vi "kalman measure step not single cycle.vi"(7 "vmax":fxp<+/-,32,0> format="%.32g", 10 "state in":T1={"pos estimate"=-30.139999389648438, "v estimate"=5.7999975979328156e-05, "weighted position error sum"=438.0, "photon count"=64, "transmit tick count"=0, "axis number"=0, "px (levels^2)"=298.0, "pxv (levels^2/ticks)"=0.003100000321865082, "pv (levels^2/ticks^2)"=6.199999802447564e-08, "vel diff (levels^2/ticks^3)"=0.0, "gx"=1.5546875, "rtwiddle"=66560.0}) -> (2 "state out":T1)   [LabVIEW 2010]
uses:
  integrating single axis kalman state.ctl
  <vilib>/rvi/FXPMathLib/FxpMul/XNode/nifxpmath_Multiplier.xnode
  <vilib>/rvi/FXPMathLib/FxpMul/subVIs/nifxpmath_Mul_SimConfig.ctl
  <vilib>/fxp/LVFixedPointQuantizationPolicyTypeDef.ctl
  <vilib>/fxp/LVFixedPointOverflowPolicyTypeDef.ctl
  <vilib>/rvi/FXPMathLib/FxpAdd/XNode/nifxpmath_Add.xnode
  <vilib>/rvi/FXPMathLib/FxpAdd/subVIs/nifxpmath_Add_SimConfig.ctl
  <vilib>/rvi/FXPMathLib/FxpReciprocal/XNode/nifxpmath_Reciprocal.xnode
  <vilib>/rvi/FXPMathLib/FxpDiv/XNode/nifxpmath_Div.xnode
  <vilib>/rvi/FXPMathLib/FxpDiv/subVIs/nifxpmath_Div_SimConfig.ctl
  <vilib>/rvi/FXPMathLib/FxpSub/XNode/nifxpmath_Sub.xnode
  <vilib>/rvi/FXPMathLib/FxpSub/subVIs/nifxpmath_Sub_SimConfig.ctl
  <vilib>/rvi/FXPMathLib/FxpMul/simVIs/DllFxpMulTemp_sub.vi
  <vilib>/rvi/FXPMathLib/FxpAdd/simVIs/DllFxpAddTemp_sub.vi
  <vilib>/rvi/FXPMathLib/FxpDiv/simVIs/DllFxpDivTemp_sub.vi
  <vilib>/rvi/FXPMathLib/FxpSub/simVIs/DllFxpSubTemp_sub.vi
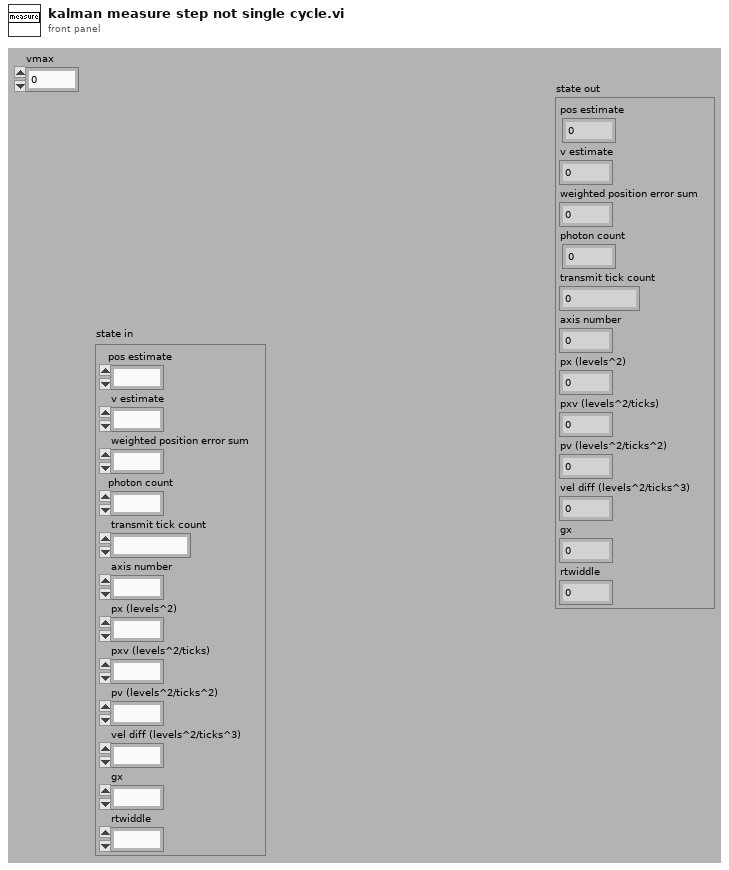
[diagram p1: front panel]
types:
  T1 = typedef "integrating single axis kalman state.ctl" = cluster{"pos estimate":fxp<+/-,32,16>, "v estimate":fxp<+/-,32,0>, "weighted position error sum":fxp<+/-,32,32>, "photon count":u32, "transmit tick count":u32, "axis number":u8, "px (levels^2)":fxp<+,32,19>, "pxv (levels^2/ticks)":fxp<+,32,2>, "pv (levels^2/ticks^2)":fxp<+,32,-14>, "vel diff (levels^2/ticks^3)":fxp<+,24,-22>, "gx":fxp<+,16,8>, "rtwiddle":fxp<+,16,26>}
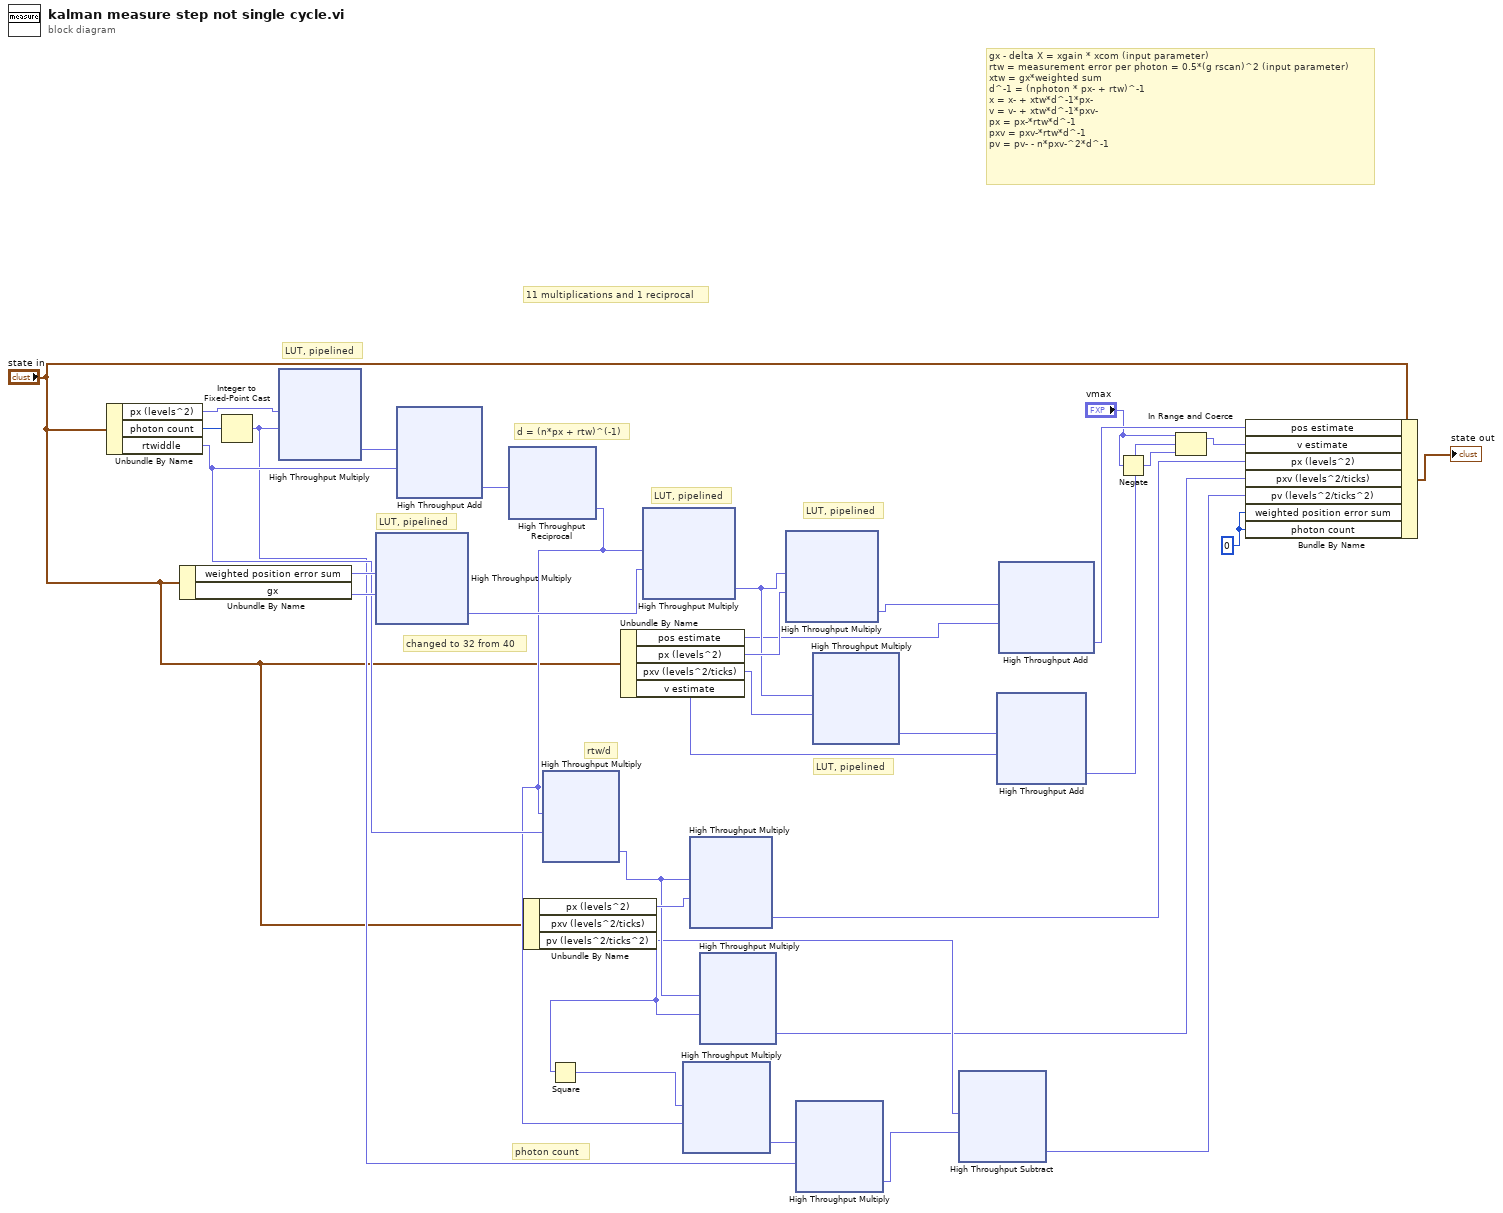
[diagram p0: block diagram]
diagram:
  w4 = i16 0
  # "LUT, pipelined"
  # "LUT, pipelined"
  # "changed to 32 from 40"
  # "LUT, pipelined"
  # "LUT, pipelined"
  # "LUT, pipelined"
  # "gx - delta X = xgain * xcom (input parameter)\nrtw = measurement error per photon = 0.5*(g rscan)^2 (input parameter)\nxtw = gx*weighted sum\nd^-1 = (nphoton * px- + rtw)^-1\nx = x- + xtw*d^-1*px-\nv = v- + xtw*d^-1*pxv-\npx = px-*rtw*d^-1\npxv = pxv-*rtw*d^-1\npv = pv- - n*pxv-^2*d^-1"
  # "11 multiplications and 1 reciprocal"
  # "photon count"
  # "rtw/d"
  # "d = (n*px + rtw)^(-1)"
  n1 = Unbundle By Name("state in") -> ("px (levels^2)"=w34:fxp<+,32,19>, "photon count"=w35:u32, "rtwiddle"=w21:fxp<+,16,26>)
  n2 = Unbundle By Name("state in") -> ("weighted position error sum"=w31:fxp<+/-,32,32>, "gx"=w30:fxp<+,16,8>)
  n3 = Integer to Fixed-Point Cast(integer=w35) -> (fixed-point=w14:fxp<+,32,32>)  [unwired: 1 in]
  n4 = xnode "High Throughput Multiply"("x"=w34, "y"=w14) -> ("x*y"=w33:fxp<+,32,42>)
  n5 = xnode "High Throughput Multiply"("x"=w31, "y"=w30) -> ("x*y"=w29:fxp<+/-,32,32>)
  n6 = xnode "High Throughput Add"("x"=w33, "y"=w21) -> ("x+y"=w32:fxp<+,32,42>)
  n7 = xnode "High Throughput Reciprocal"("x"=w32) -> ("1/x"=w16:fxp<+,32,-10>)
  n8 = Unbundle By Name("state in") -> ("px (levels^2)"=w20:fxp<+,32,19>, "pxv (levels^2/ticks)"=w18:fxp<+,32,2>, "pv (levels^2/ticks^2)"=w13:fxp<+,32,-14>)
  n9 = xnode "High Throughput Multiply"("x"=w16, "y"=w21) -> ("x*y"=w19:fxp<+,32,0>)
  n10 = Square(x=w18) -> (x^2=w17:fxp<+,32,4>)
  n11 = Unbundle By Name("state in") -> ("pos estimate"=w23:fxp<+/-,32,16>, "px (levels^2)"=w28:fxp<+,32,19>, "pxv (levels^2/ticks)"=w26:fxp<+,32,2>, "v estimate"=w22:fxp<+/-,32,0>)
  n12 = xnode "High Throughput Multiply"("x"=w16, "y"=w29) -> ("x*y"=w27:fxp<+/-,32,11>)
  n13 = xnode "High Throughput Multiply"("x"=w17, "y"=w16) -> ("x*y"=w15:fxp<+,32,-14>)
  n14 = xnode "High Throughput Multiply"("x"=w19, "y"=w20) -> ("x*y"=w8:fxp<+,32,19>)
  n15 = xnode "High Throughput Multiply"("x"=w19, "y"=w18) -> ("x*y"=w7:fxp<+,32,2>)
  n16 = xnode "High Throughput Multiply"("x"=w27, "y"=w28) -> ("x*y"=w24:fxp<+/-,32,16>)
  n17 = xnode "High Throughput Multiply"("x"=w15, "y"=w14) -> ("x*y"=w12:fxp<+,32,-14>)
  n18 = xnode "High Throughput Multiply"("x"=w27, "y"=w26) -> ("x*y"=w25:fxp<+/-,32,0>)
  n19 = xnode "High Throughput Subtract"("x"=w13, "y"=w12) -> ("x-y"=w6:fxp<+,32,-14>)
  n20 = xnode "High Throughput Add"("x"=w25, "y"=w22) -> ("x+y"=w9:fxp<+/-,32,0>)
  n21 = xnode "High Throughput Add"("x"=w24, "y"=w23) -> ("x+y"=w10:fxp<+/-,32,16>)
  n22 = Negate(x="vmax") -> (-x=w1:fxp<+/-,32,0>)
  n23 = In Range and Coerce(upper limit="vmax", x=w9, lower limit=w1) -> (coerced(x)=w3:fxp<+/-,32,0>)  [unwired: 1 out]
  n24 = Bundle By Name(cluster="state in", "pos estimate"=w10, "v estimate"=w3, "px (levels^2)"=w8, "pxv (levels^2/ticks)"=w7, "pv (levels^2/ticks^2)"=w6, "weighted position error sum"=w4, "photon count"=w4) -> (→"state out":T1)
